vi "Get Table Names.vi"(7 "Sheet Name":string, 8 "error in":errorcluster, 11 "SpreadsheetDoc in":refnum<k24>) -> (0 "error out":errorcluster, 2 "Table Names":string[](array[string]), 3 "SpreadsheetDoc out":refnum<k24>, 5 "Sheet Name":string)   [LabVIEW 2019, in "Open Xml.lvlib"]
uses:
  Open Xml.lvlib
  D:/git/Open-Xml-LabVIEW/Source/DocumentFormat.OpenXml.dll
  DocumentFormat.OpenXml.dll
  D:/git/Open-Xml-LabVIEW/Source/DocumentFormat.OpenXml.Framework.dll
  DocumentFormat.OpenXml.Framework.dll
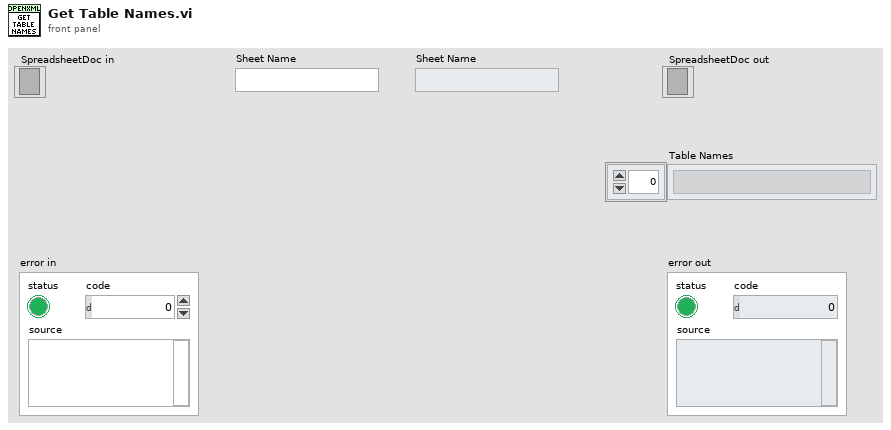
[diagram p1: front panel]
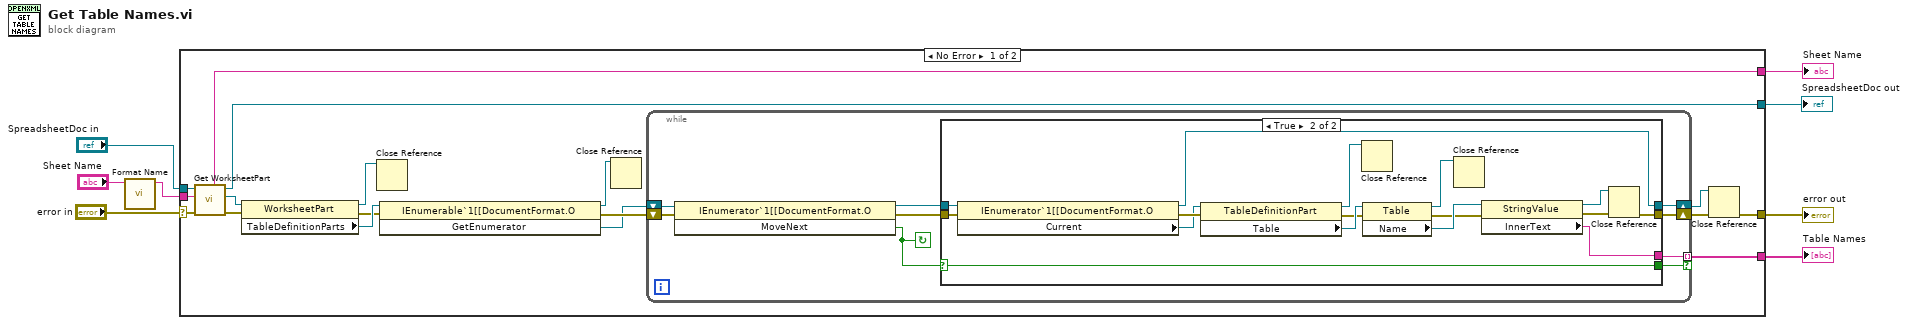
[diagram p0: block diagram]
diagram:
  n1 = call "Format Name.vi"("Sheet Name"="Sheet Name") -> ("Formatted Sheet Name"=w2:string)  [unwired: 10 in]
  n2 = case shown="No Error" "error in" {
    selector: "error in" -> [w25 w55]
    tunnel: "SpreadsheetDoc in" -> [w24 w54]
    tunnel: [w23 _] -> w5
    tunnel: [w21 w54] -> w4
    tunnel: [w18 w55] -> w3
    tunnel: w2 -> [w16 _]
    tunnel: [w10 _] -> w1
    frame No Error {
      n3 = call "Get WorksheetPart.vi"("error in"=w25, "Sheet Name"=w16, "SpreadsheetDoc in"=w24) -> ("error out"=w20:errorcluster, "WorksheetPart"=w22:refnum<k24>, "SpreadsheetDoc out"=w21:refnum<k24>, "SheetName"=w23:string)  [unwired: 5 in]
      n4 = property class="WorksheetPart"(reference=w22, error in=w20) -> (reference out=w9:refnum<k24>, error out=w14:errorcluster, "TableDefinitionParts"=w15:refnum<k24>)
      n5 = Close Reference(reference=w9) -> ()  [unwired: 1 in, 1 out]
      n6 = invoke class="IEnumerable`1[[DocumentFormat.O" method="GetEnumerator"(reference=w15, error in=w14) -> (reference out=w11:refnum<k24>, error out=w13:errorcluster, "GetEnumerator"=w12:refnum<k24>)  [unwired: 1 in]
      n7 = Close Reference(reference=w11) -> ()  [unwired: 1 in, 1 out]
      n8 = while {
        shift-right: [w33] -> w17
        shift-left: w12 -> [w30]
        shift-right: [w28] -> w19
        shift-left: w13 -> [w34]
        tunnel: [w32] -> w10 mode=indexing if=w26
        stop <- w27 continue-if-true
        n9 = invoke class="IEnumerator`1[[DocumentFormat.O" method="MoveNext"(reference=w30, error in=w34) -> (reference out=w29:refnum<k24>, error out=w31:errorcluster, "MoveNext"=w27:bool)  [unwired: 1 in]
        n10 = case shown="True" w27 {
          selector: w27 -> [w35 w38]
          tunnel: [w36 w47] -> w33
          tunnel: [_ w46] -> w32
          tunnel: w31 -> [w37 w43]
          tunnel: w29 -> [w36 w42]
          tunnel: [w37 w39] -> w28
          tunnel: [w35 w38] -> w26
          frame False {
          }
          frame True {
            n11 = property class="IEnumerator`1[[DocumentFormat.O"(reference=w42, error in=w43) -> (reference out=w47:refnum<k24>, error out=w49:errorcluster, "Current"=w48:refnum<k24>)
            n12 = property class="TableDefinitionPart"(reference=w48, error in=w49) -> (reference out=w50:refnum<k24>, error out=w51:errorcluster, "Table"=w53:refnum<k24>)
            n13 = Close Reference(reference=w50) -> ()  [unwired: 1 in, 1 out]
            n14 = property class="Table"(reference=w53, error in=w51) -> (reference out=w44:refnum<k24>, error out=w41:errorcluster, "Name"=w52:refnum<k24>)
            n15 = Close Reference(reference=w44) -> ()  [unwired: 1 in, 1 out]
            n16 = property class="StringValue"(reference=w52, error in=w41) -> (reference out=w45:refnum<k24>, error out=w40:errorcluster, "InnerText"=w46:string)
            n17 = Close Reference(reference=w45, error in (no error)=w40) -> (error out=w39:errorcluster)
          }
        }
      }
      n18 = Close Reference(reference=w17, error in (no error)=w19) -> (error out=w18:errorcluster)
    }
    frame Error {
    }
  }
  "SpreadsheetDoc out" <- w4
  "Table Names" <- w1
  "error out" <- w3
  "Sheet Name" <- w5
